vi "Deadband_Filter.vi"(9 "Range":dbl=25.0 format="%#_13g", 10 "Target":dbl format="%#_13g", 11 "Joystick Input":dbl format="%#_13g") -> (3 "Output":dbl)   [LabVIEW 2016]
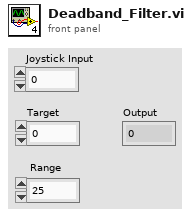
[diagram p1: front panel]
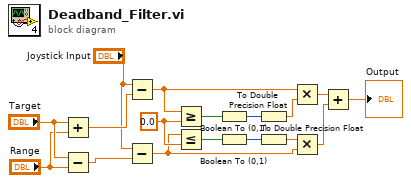
[diagram p0: block diagram]
diagram:
  w17 = 0.0
  n1 = Add(x="Target", y="Range") -> (x+y=w4:dbl)
  n2 = Subtract(x="Target", y="Range") -> (x-y=w3:dbl)
  n3 = Subtract(x="Joystick Input", y=w4) -> (x-y=w15:dbl)
  n4 = Subtract(x="Joystick Input", y=w3) -> (x-y=w13:dbl)
  n5 = Greater Or Equal?(x=w15, y=w17) -> (x >= y?=w8:bool)
  n6 = Less Or Equal?(x=w13, y=w17) -> (x <= y?=w10:bool)
  n7 = Boolean To (0,1)(Boolean=w8) -> (0, 1=w7:i16)
  n8 = Boolean To (0,1)(Boolean=w10) -> (0, 1=w9:i16)
  n9 = To Double Precision Float(number=w7) -> (double precision float=w16:dbl)
  n10 = To Double Precision Float(number=w9) -> (double precision float=w14:dbl)
  n11 = Multiply(x=w15, y=w16) -> (x*y=w12:dbl)
  n12 = Multiply(x=w14, y=w13) -> (x*y=w11:dbl)
  n13 = Add(x=w12, y=w11) -> (x+y=→"Output":dbl)
